vi "GLdrv_TRIG_COND_LOGI.vi"(0 "Connection ID":T1, 5 "COND":i32=1 min=0 max=1, 7 "Logic CH":i32=1 min=1, 9 "Set":enum16{"OFF", "HI", "LO"}(ring), 11 "error in (no error)":errorcluster, 13 "Query(f)":bool) -> (4 "Connection ID Out":T1, 10 "Set out":enum16{"OFF", "HI", "LO"}(ring), 15 "error out":errorcluster)   [LabVIEW 2017, in "GL860_Driver.lvlib"]
doc: "ロジックCHのトリガ種類を設定します\nOFF：　ロジックCHのトリガをOffにします\nHI：　ロジックCHのトリガをハイパターンに設定します\nLO：　ロジックCHのトリガをローパターンに設定します\n例）　:TRIG:COND0:LOGI1:SET HI (ロジックCH1のスタートトリガをHI\nに設定します)\n※ロジックは16CH単位のパターン合致検知です。"
uses:
  GL860_Driver.lvlib
  ConnectionID.ctl
  GLdrv_RW.ctl
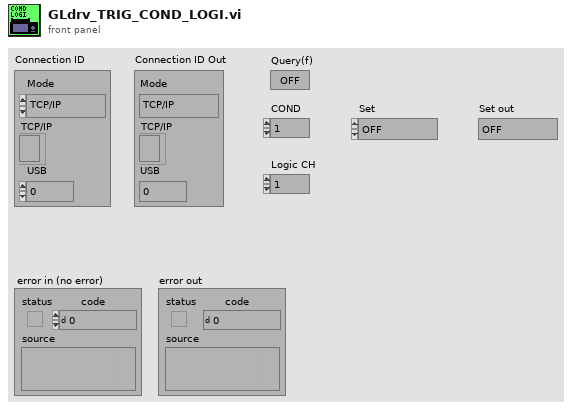
[diagram p1: front panel]
types:
  T1 = typedef "ConnectionID.ctl" = cluster{"Mode":enum16{"TCP/IP", "USB"}, "TCP/IP":refnum<k5>, "USB":i32}
  T2 = typedef "GLdrv_RW.ctl" = enum16{"Auto", "Read", "Write", "Buffer"}
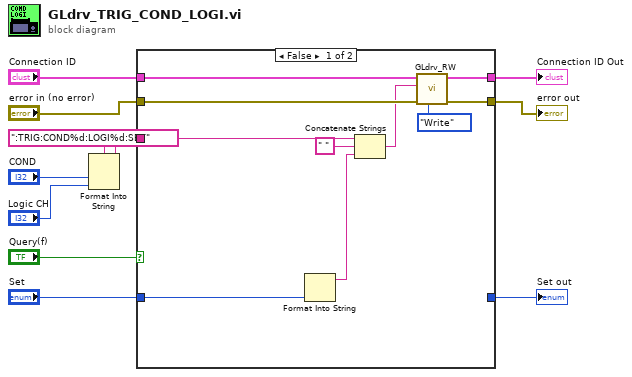
[diagram p0: block diagram]
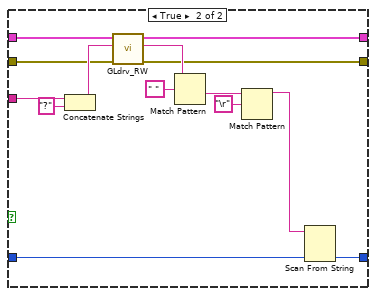
[diagram p2: hidden frame]
diagram:
  n1 = Format Into String(format string=":TRIG:COND%d:LOGI%d:SET" ("Command"), "COND", "Logic CH") -> (resulting string=w6:string)  [unwired: 2 in, 1 out]
  n2 = case shown="FALSE" "Query(f)" {
    tunnel: w6 -> [w21 w32]
    tunnel: [w16 w24] -> w11
    tunnel: [w18 w28] -> w10
    tunnel: "Connection ID" -> [w19 w29]
    tunnel: "error in (no error)" -> [w17 w25]
    tunnel: "Set" -> [w12 w23]
    tunnel: [_ w22] -> w4
    frame False {
      n3 = Format Into String(w12) -> (resulting string=w13:string)  [unwired: 3 in, 1 out]
      n4 = Concatenate Strings(w21, " " ("string"), w13) -> (w15:string)
      n5 = call "GLdrv_RW.vi"("Mode(read)"=GLdrv_RW."Write", "error in (no error)"=w17, "data in"=w15, "Connection ID"=w19) -> ("error out"=w16:errorcluster, "Connection ID Out"=w18:T1)  [unwired: 3 in, 3 out]
    }
    frame True {
      n6 = Concatenate Strings(w32, "?" ("string")) -> (w27:string)
      n7 = call "GLdrv_RW.vi"("error in (no error)"=w25, "data in"=w27, "Connection ID"=w29) -> ("error out"=w24:errorcluster, "data out"=w26:string, "Connection ID Out"=w28:T1)  [unwired: 4 in, 2 out]
      n8 = Match Pattern(string=w26, regular expression=" " ("search string/char (-)")) -> (after substring=w33:string)  [unwired: 4 out]
      n9 = Match Pattern(string=w33, regular expression="\r") -> (before substring=w30:string)  [unwired: 4 out]
      n10 = Scan From String(input string=w30, default 1=w23) -> (output 1=w22:enum16{"OFF", "HI", "LO"})  [unwired: 3 in, 3 out]
    }
  }
  "Connection ID Out" <- w10
  "error out" <- w11
  "Set out" <- w4
